vi "Init.vi"(8 "error in (no error)":errorcluster, 10 "srvPort":i32=851, 11 "srvAddress (\"\"=local)":string) -> (0 "error out":errorcluster, 3 "TCatAdsNet":refnum<class "AdsNET.lvclass">)   [LabVIEW 2016, in "TCatAdsNet.lvlib" / "AdsNET.lvclass"]
doc: "Instance class data. For a local ADS server, the address must be empty string."
uses:
  AdsNET.lvclass
  AdsNET.lvclass/AdsNET.ctl
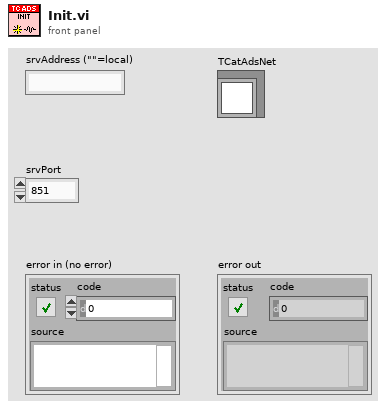
[diagram p1: front panel]
types:
  T1 = cluster{"Name":string, "IndexGroup":i64, "IndexOffset":i64, "Size":i32, "Type":string, "Datatype":i32, "Comment":string}[]
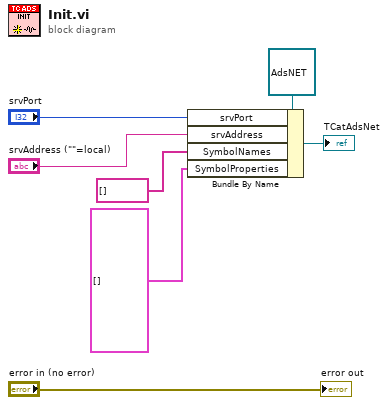
[diagram p0: block diagram]
diagram:
  n1 = Bundle By Name(cluster=refnum<class "AdsNET.lvclass"> refnum ("TCatAdsNet.lvlib:AdsNET.lvclass"), "srvPort"="srvPort", "srvAddress"="srvAddress (\"\"=local)", "SymbolNames"=string[] [], "SymbolProperties"=T1 []) -> (→"TCatAdsNet":refnum<class "AdsNET.lvclass">)
  "error out" <- "error in (no error)"
